vi "Configure Channel Label.vi"(7 "Enable Label (T: Enable)":bool=TRUE, 8 "error in (no error)":errorcluster, 9 "Label (\"Test\")":string="Test", 10 "Channel Name (0: Channel 1)":u16(ring) items=["Channel 1", "Channel 2", "Channel 3", "Channel 4", "DIG 0", "DIG 1", "DIG 2", "DIG 3", "DIG 4", "DIG 5", "DIG 6", "DIG 7", "DIG 8", "DIG 9", "DIG 10", "DIG 11", "DIG 12", "DIG 13", "DIG 14", "DIG 15"], 11 "VISA resource name":refnum<visa-resource-name>) -> (0 "error out":errorcluster, 3 "VISA resource name out":refnum<visa-resource-name>)   [LabVIEW 2017, in "Agilent 6000 Series.lvlib"]
doc: "This VI sets the analog or digital channel label."
uses:
  <instrlib>/Agilent 6000 Series/Agilent 6000 Series.lvlib
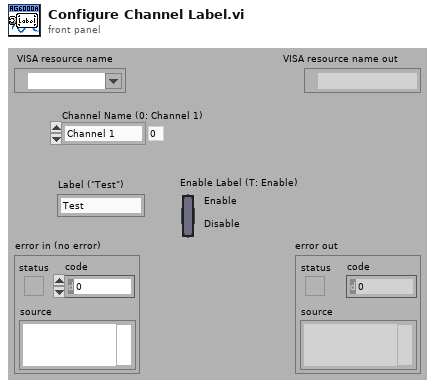
[diagram p1: front panel]
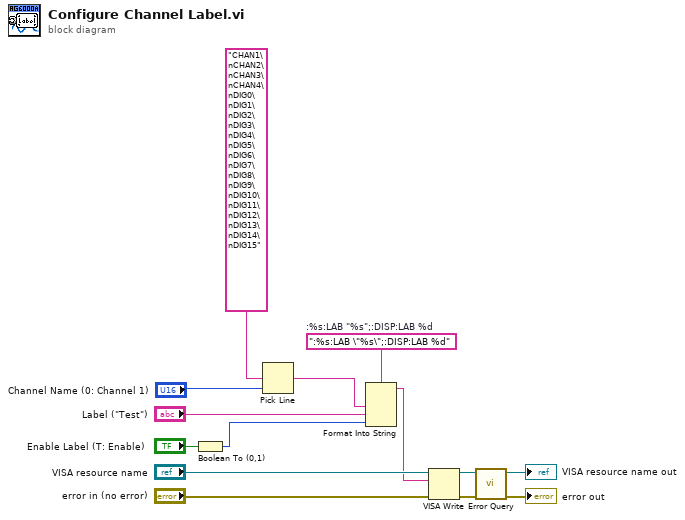
[diagram p0: block diagram]
diagram:
  w8 = ":%s:LAB \"%s\";:DISP:LAB %d"  # :%s:LAB "%s";:DISP:LAB %d
  n1 = Boolean To (0,1)(Boolean="Enable Label (T: Enable)") -> (0, 1=w2:i16)
  n2 = Pick Line(multi-line string="CHAN1\nCHAN2\nCHAN3\nCHAN4\nDIG0\nDIG1\nDIG2\nDIG3\nDIG4\nDIG5\nDIG6\nDIG7\nDIG8\nDIG9\nDIG10\nDIG11\nDIG12\nDIG13\nDIG14\nDIG15", line index="Channel Name (0: Channel 1)") -> (output string=w5:string)  [unwired: 1 in]
  n3 = Format Into String(format string=w8, w5, "Label (\"Test\")", w2) -> (resulting string=w7:string)  [unwired: 2 in, 1 out]
  n4 = VISA Write(VISA resource name="VISA resource name", write buffer=w7, error in (no error)="error in (no error)") -> (VISA resource name out=w10:refnum<visa-resource-name>, error out=w9:errorcluster)  [unwired: 1 out]
  n5 = call <instrlib>:"Error Query.vi"("error in (no error)"=w9, "VISA resource name"=w10) -> ("error out"=→"error out":errorcluster, "VISA resource name out"=→"VISA resource name out":refnum<visa-resource-name>)  [unwired: 6 in, 2 out]
